vi "Configure Display.vi"(0 "VISA resource name (in)":refnum<visa-resource-name>, 1 "Decimal Point (F.FFF)":T4, 2 "Temperature Units (none)":T3, 3 "Display Color (GREEN)":T2, 4 "Display Brightness (LOW)":T1, 5 "error in (no error)":errorcluster, 6 "Unit Address (-1)":i32=-1, 8 "Retry Attempts (0)":i32 min=0) -> (14 "VISA resource name (out)":refnum<visa-resource-name>, 16 "Response Cluster":T5 {"Command ID" format="%x"}, 19 "error out":errorcluster)   [LabVIEW 2020, in "Omega Platinum Series.lvlib"]
doc: "Configures the display for the controller."
uses:
  <instrlib>/RxnRover/OmegaPlatinumSeriesDriver/Omega Platinum Series.lvlib
  <instrlib>/RxnRover/OmegaPlatinumSeriesDriver/Public/Type Defs/Response.ctl
  <instrlib>/RxnRover/OmegaPlatinumSeriesDriver/Public/Type Defs/Display Decimal Point.ctl
  <instrlib>/RxnRover/OmegaPlatinumSeriesDriver/Public/Type Defs/Display Temperature Units.ctl
  <instrlib>/RxnRover/OmegaPlatinumSeriesDriver/Public/Type Defs/Display Color.ctl
  <instrlib>/RxnRover/OmegaPlatinumSeriesDriver/Public/Type Defs/Display Brightness.ctl
panel:
  out "Command":string
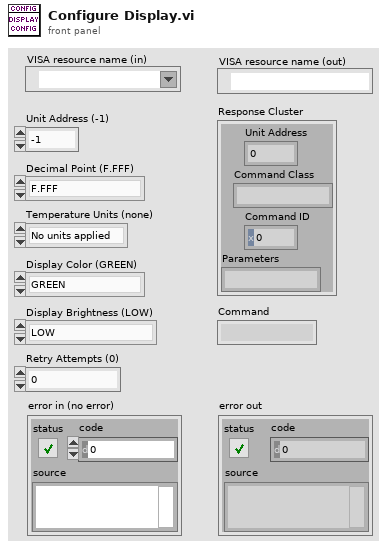
[diagram p1: front panel]
types:
  T1 = typedef "Omega Platinum Series.lvlib/Display Brightness.ctl" = enum16{"LOW", "MEDIUM", "HIGH"}
  T2 = typedef "Omega Platinum Series.lvlib/Display Color.ctl" = enum16{"GREEN", "RED", "AMBER"}
  T3 = typedef "Omega Platinum Series.lvlib/Display Temperature Units.ctl" = enum16{"No units applied", "Celsius", "Fahrenheit"}
  T4 = typedef "Omega Platinum Series.lvlib/Display Decimal Point.ctl" = enum16{"F.FFF", "FF.FF"}
  T5 = typedef "Omega Platinum Series.lvlib/Response.ctl" = cluster{"Unit Address":i32, "Command Class":string, "Command ID":u32, "Parameters":string}
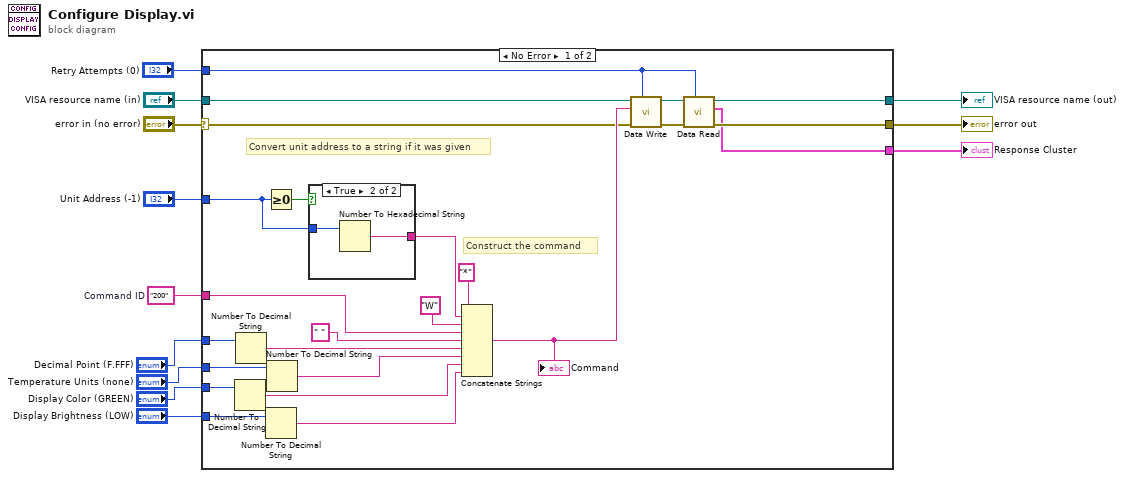
[diagram p0: block diagram]
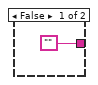
[diagram p2: hidden frame]
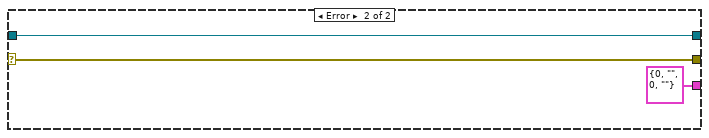
[diagram p3: hidden frame]
diagram:
  w12 = "200"  # Command ID
  n1 = case shown="No Error" "error in (no error)" {
    selector: "error in (no error)" -> [w30 w42]
    tunnel: w12 -> [w23 _]
    tunnel: "Unit Address (-1)" -> [w34 _]
    tunnel: [w26 w42] -> w9
    tunnel: "VISA resource name (in)" -> [w32 w41]
    tunnel: [w27 w41] -> w7
    tunnel: [w25 T5 {"Unit Address"=0, "Command Class"="", "Command ID"=0, "Parameters"=""} ("Response Cluster")] -> w6
    tunnel: "Decimal Point (F.FFF)" -> [w20 _]
    tunnel: "Temperature Units (none)" -> [w19 _]
    tunnel: "Display Color (GREEN)" -> [w18 _]
    tunnel: "Display Brightness (LOW)" -> [w17 _]
    tunnel: "Retry Attempts (0)" -> [w13 _]
    frame No Error {
      # "Convert unit address to a string if it was given"
      # "Construct the command"
      n2 = Number To Decimal String(number=w18) -> (decimal integer string=w15:string)  [unwired: 1 in]
      n3 = Number To Decimal String(number=w20) -> (decimal integer string=w22:string)  [unwired: 1 in]
      n4 = Greater Or Equal To 0?(x=w34) -> (x >= 0?=w36:bool)
      n5 = Number To Decimal String(number=w17) -> (decimal integer string=w16:string)  [unwired: 1 in]
      n6 = Number To Decimal String(number=w19) -> (decimal integer string=w14:string)  [unwired: 1 in]
      n7 = case shown="True" w36 {
        tunnel: w34 -> [_ w39]
        tunnel: ["" w38] -> w33
        frame False {
        }
        frame True {
          n8 = Number To Hexadecimal String(2:w39) -> (0:w38:string)  [unwired: 1 in]
        }
      }
      n9 = Concatenate Strings("*" ("string"), w33, "W" ("string"), w23, " " ("string"), w22, w14, w15, w16) -> (w31:string)
      "Command" <- w31
      n10 = call <instrlib>:"Data Write.vi"("Retry Attempts (0)"=w13, "error in (no error)"=w30, "Command"=w31, "VISA Refnum in"=w32) -> ("error out"=w29:errorcluster, "VISA Refnum out"=w28:refnum<visa-resource-name>)  [unwired: 6 in]
      n11 = call <instrlib>:"Data Read.vi"("Retry Attempts (0)"=w13, "error in (no error)"=w29, "VISA Refnum in"=w28) -> ("error out"=w26:errorcluster, "Response Cluster"=w25:T5, "VISA Refnum out"=w27:refnum<visa-resource-name>)  [unwired: 5 in, 1 out]
    }
    frame Error {
    }
  }
  "error out" <- w9
  "VISA resource name (out)" <- w7
  "Response Cluster" <- w6
